vi "Find&Exchange_dots_ID-6.vi"(4 "Track ID Arr IN":u16[](array[numeric]), 5 "Dot matrix (stat)":i16[][](array[numeric]), 6 "track ID IN":u16, 7 "(X,Y...) Tracks":dbl[][](array[numeric]), 8 "error IN":errorcluster, 9 "frame (col)":i32, 10 "index of \ndot in frame":i32, 11 "ID-dot matrix":u16[][](array[numeric])) -> (0 "error OUT":errorcluster, 1 "track ID OUT":u16, 2 "Track ID Arr OUT":u16[](array[numeric]), 3 "ID-dot matrix OUT":u16[][](array[numeric]))   [LabVIEW 2013]
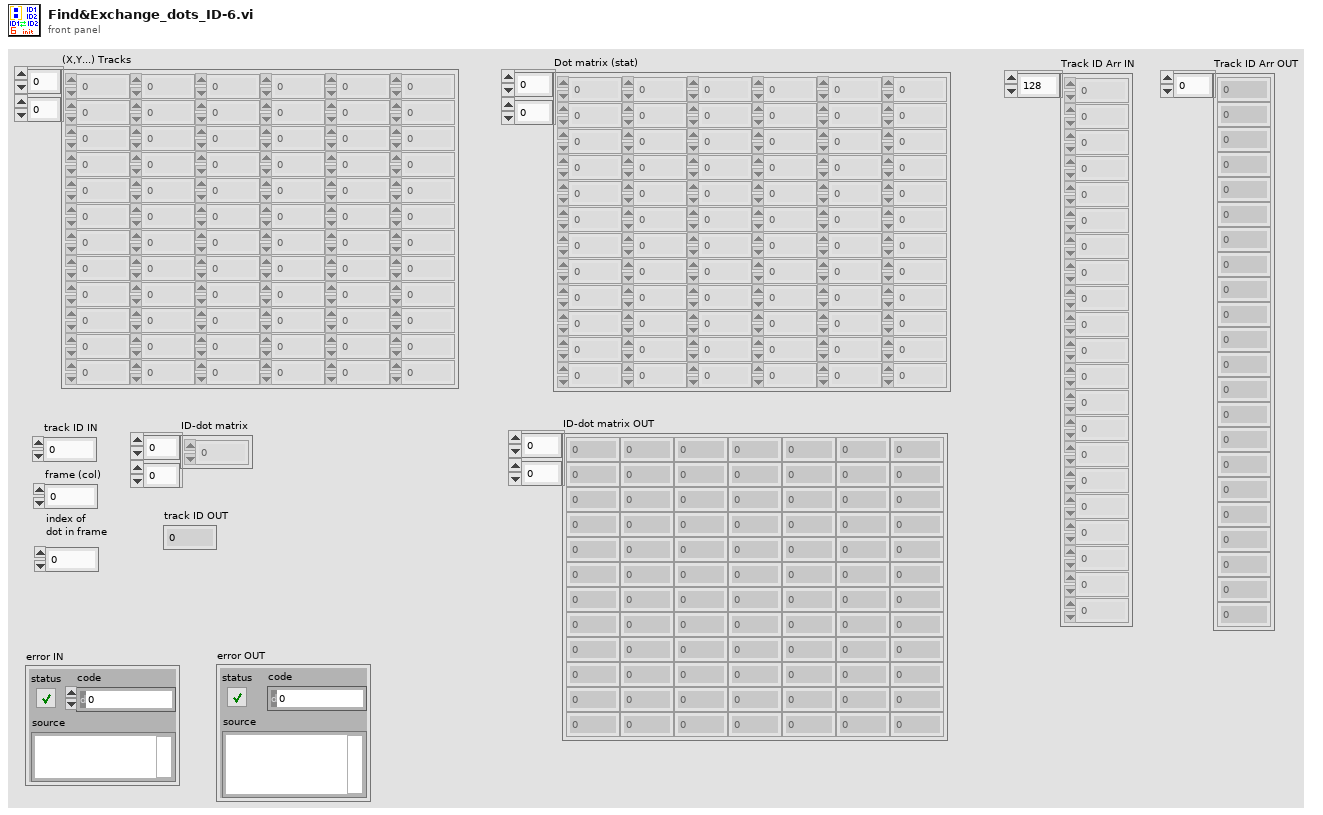
[diagram p1: front panel]
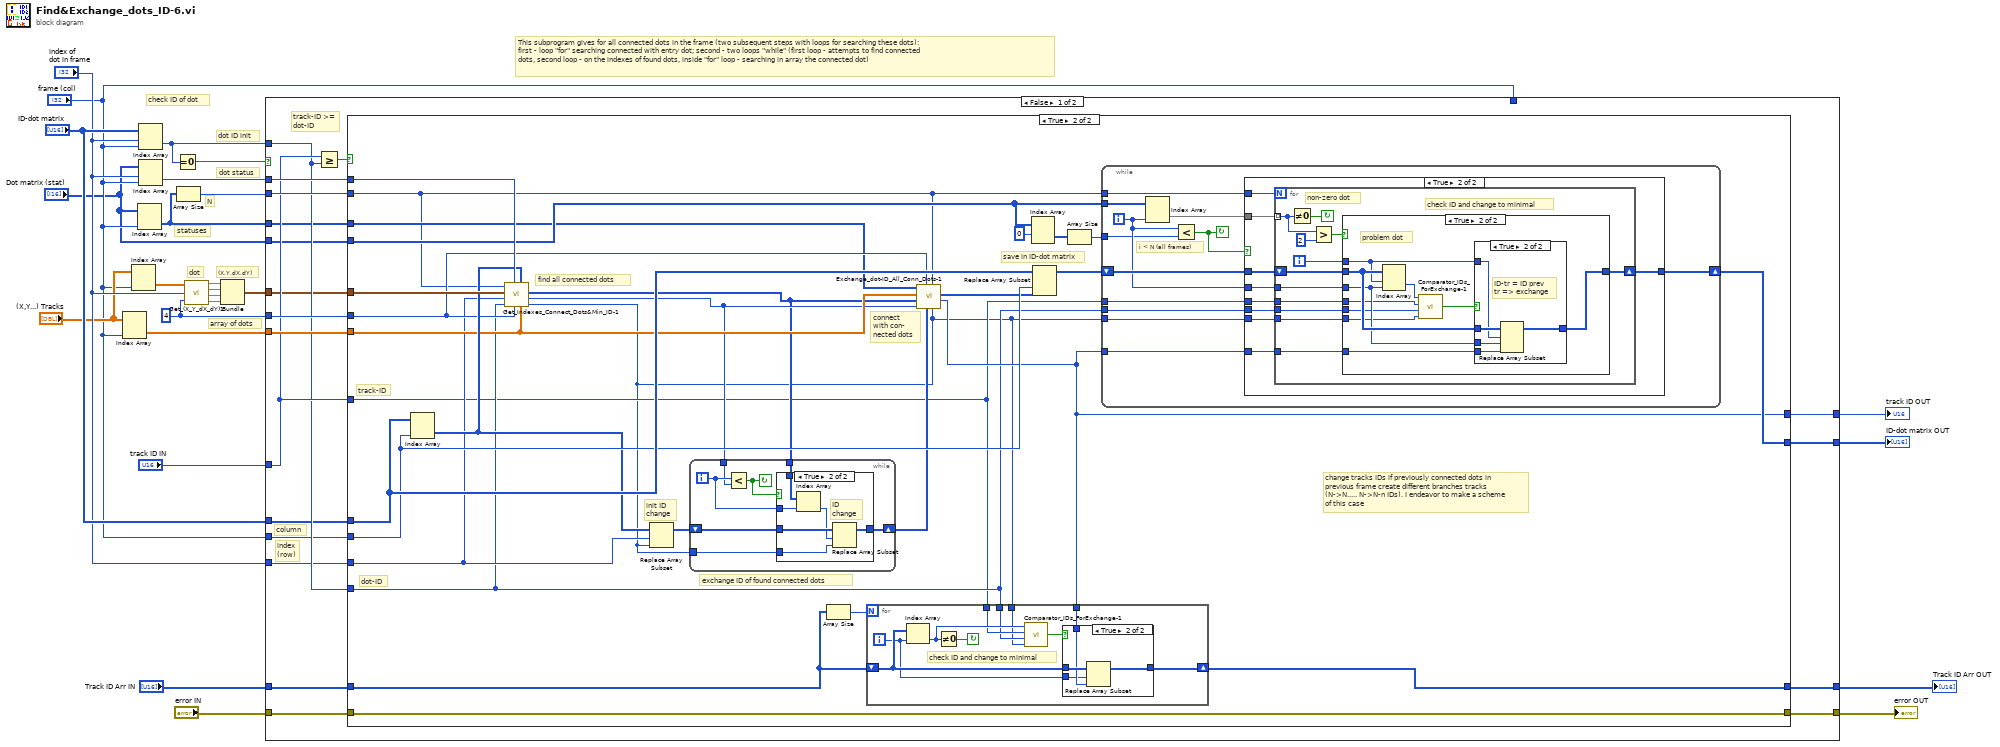
[diagram p0: block diagram]
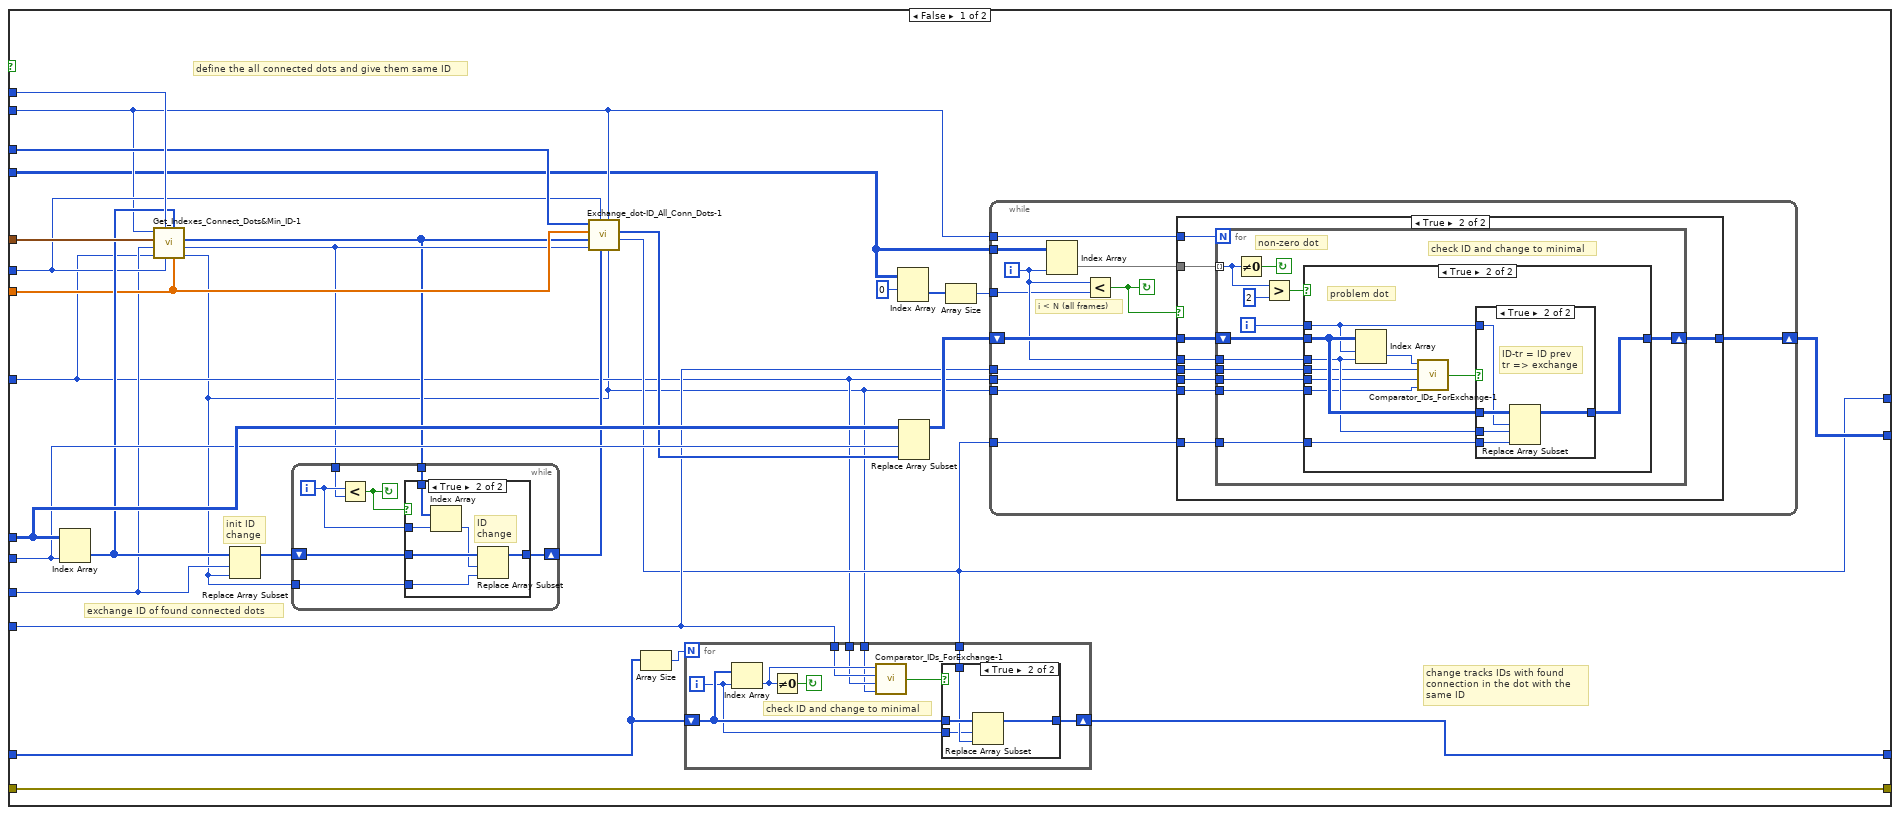
[diagram p2: hidden frame]
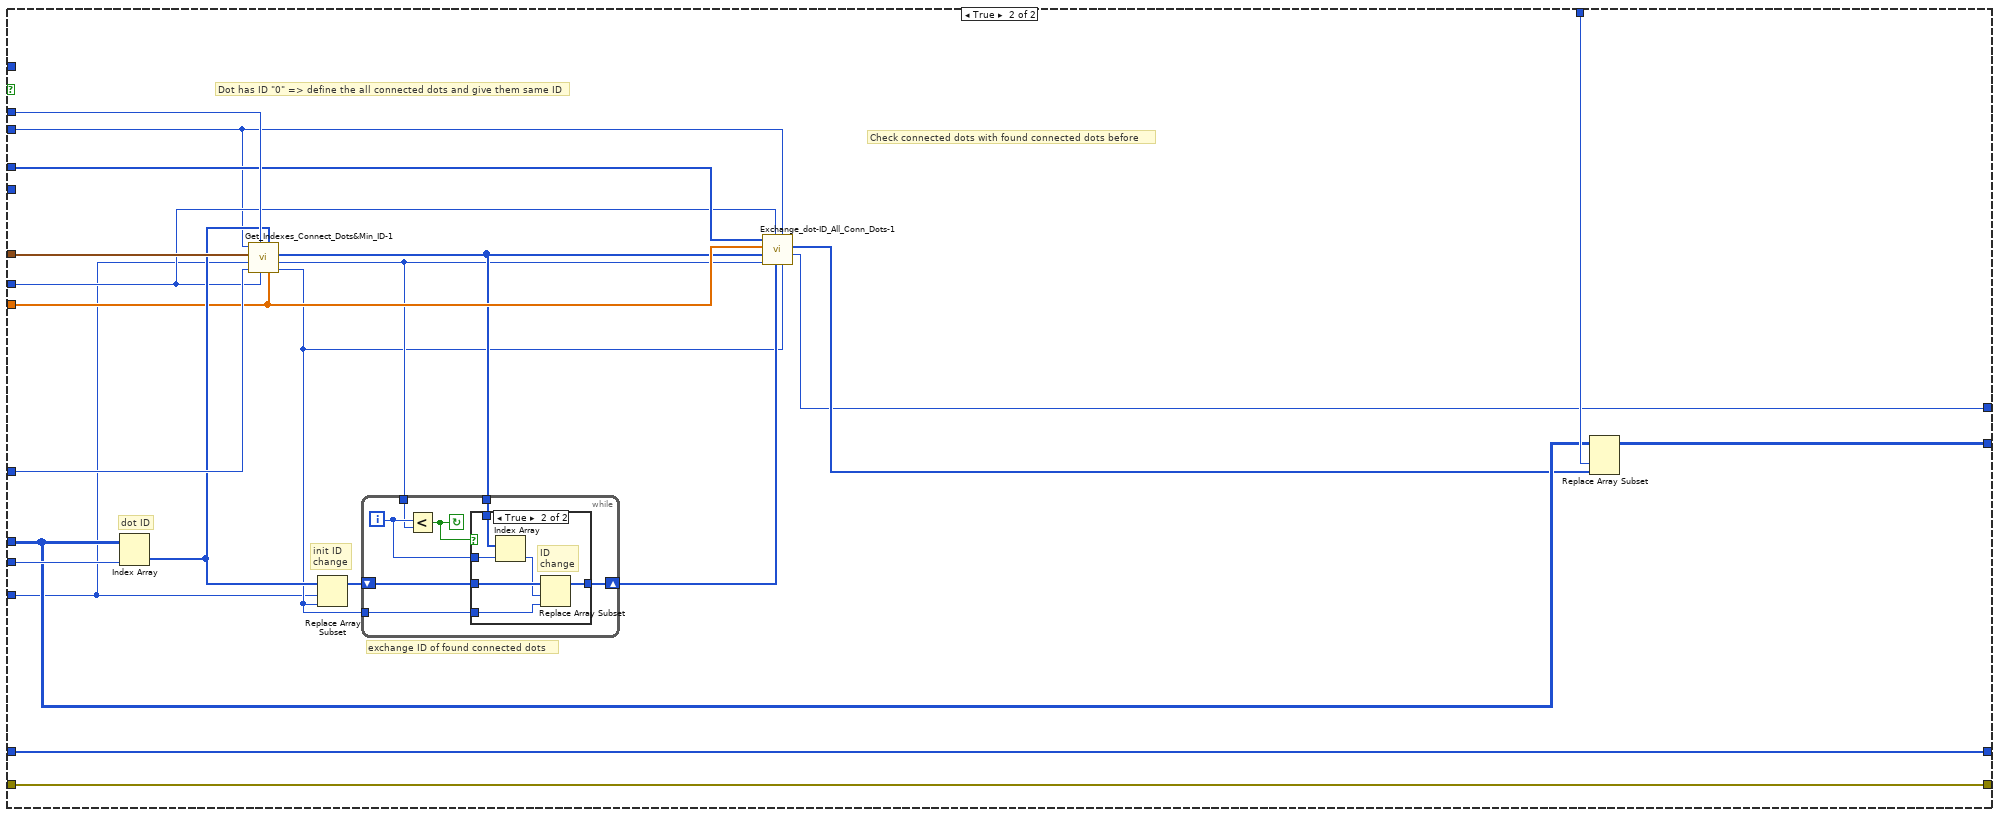
[diagram p13: hidden frame]
diagram:
  w19 = 4 ("multiplier")
  # "array of dots"
  # "dot ID init"
  # "dot status"
  # "(X,Y,dX,dY)"
  # "N"
  # "statuses"
  # "This subprogram gives for all connected dots in the frame (two subsequent steps with loops for searching these dots): \nfirst - loop \"for\" searching connected with entry dot; second - two loops \"while\" (first loop - attempts to find connected \ndots, second loop - on the indexes of found dots, inside \"for\" loop - searching in array the connected dot)"
  # "dot"
  # "check ID of dot"
  n1 = Index Array(array="(X,Y...) Tracks", index (col)="frame (col)") -> (element=w23:dbl[])  [unwired: 1 in]
  n2 = Index Array(array="(X,Y...) Tracks", index (col)="frame (col)") -> (element=w20:dbl[])  [unwired: 1 in]
  n3 = Index Array(array="Dot matrix (stat)", index (col)="frame (col)") -> (element=w24:i16[])  [unwired: 1 in]
  n4 = Index Array(array="ID-dot matrix", index (row)="index of \ndot in frame", index (col)="frame (col)") -> (element=w16:u16)
  n5 = Index Array(array="Dot matrix (stat)", index (row)="index of \ndot in frame", index (col)="frame (col)") -> (element=w22:i16)
  n6 = Equal To 0?(x=w16) -> (x = 0?=w21:bool)
  n7 = Array Size(array=w24) -> (size(s)=w25:i32)
  n8 = call "Get_(X_Y_dX_dY)1.vi"("(X,Y,dX,dY)"=w20, "index"="index of \ndot in frame", "multiplier"=w19) -> ("X"=w6:dbl, "Y"=w5:dbl, "dX"=w4:dbl, "dY"=w3:dbl)
  n9 = Bundle("X"=w6, "Y"=w5, "dX"=w4, "dY"=w3) -> (w2:cluster{"X":dbl, "Y":dbl, "dX":dbl, "dY":dbl})  [unwired: 1 in]
  n10 = case shown="False" w21 {
    tunnel: w25 -> [w39 w271]
    tunnel: w24 -> [w26 w273]
    tunnel: w23 -> [w38 w270]
    tunnel: w22 -> [w36 w276]
    tunnel: w19 -> [w37 w272]
    tunnel: "ID-dot matrix" -> [w32 w279]
    tunnel: "frame (col)" -> [w30 w280]
    tunnel: "index of \ndot in frame" -> [w28 w263]
    tunnel: "track ID IN" -> [w35 w275]
    tunnel: w16 -> [w34 _]
    tunnel: "error IN" -> [w43 w284]
    tunnel: [w42 w284] -> w13
    tunnel: [w41 w264] -> w12
    tunnel: [w31 w282] -> w11
    tunnel: "Track ID Arr IN" -> [w29 w281]
    tunnel: [w40 w281] -> w9
    tunnel: "frame (col)" -> [_ w283]
    tunnel: "Dot matrix (stat)" -> [w33 _]
    tunnel: w2 -> [w27 w277]
    frame False {
      # "column"
      # "index\n(row)"
      # "track-ID >=\ndot-ID"
      n11 = Greater Or Equal?(x=w35, y=w34) -> (x >= y?=w44:bool)
      n12 = case shown="True" w44 {
        tunnel: [w48 w166] -> w41
        tunnel: w34 -> [w50 w156]
        tunnel: w35 -> [w46 w155]
        tunnel: w43 -> [w71 w182]
        tunnel: [w71 w182] -> w42
        tunnel: w29 -> [w72 w180]
        tunnel: [w47 w179] -> w40
        tunnel: w39 -> [w52 w162]
        tunnel: w38 -> [w64 w164]
        tunnel: w37 -> [w63 w165]
        tunnel: w36 -> [w67 w173]
        tunnel: w33 -> [w51 w171]
        tunnel: w32 -> [w70 w178]
        tunnel: w30 -> [w69 w176]
        tunnel: [w49 w175] -> w31
        tunnel: w28 -> [w61 w161]
        tunnel: w27 -> [w68 w174]
        tunnel: w26 -> [w65 w163]
        frame False {
          # "define the all connected dots and give them same ID"
          # "init ID\nchange"
          # "exchange ID of found connected dots"
          # "change tracks IDs with found \nconnection in the dot with the \nsame ID"
          n13 = Index Array(array=w70, index (col)=w69) -> (element=w66:u16[])  [unwired: 1 in]
          n14 = call "Get_Indexes_Connect_Dots&Min_ID-1.vi"("(X,Y...) Tracks col"=w64, "ID-dot col"=w66, "multiplier (x4)"=w63, "dot status"=w67, "initial ID"=w46, "Current Dot \nindex"=w61, "Dot coord"=w68, "N elem. in col"=w52) -> ("minimal ID \nbetween them"=w45:u16, "amount"=w59:i32, "Indexex Connec\ndots"=w58:i32[])  [unwired: 1 in]
          n15 = Replace Array Subset(array=w66, new element=w45, index=w61) -> (w60:u16[])
          n16 = while {
            shift-right: [w129] -> w57
            shift-left: w60 -> [w128]
            tunnel: w45 -> [w127]
            tunnel: w59 -> [w125]
            tunnel: w58 -> [w130]
            i -> [w126]
            stop <- w131 continue-if-true
            n17 = Less?(x=w126, y=w125) -> (x < y?=w131:bool)
            n18 = case shown="True" w131 {
              tunnel: w130 -> [_ w138]
              tunnel: w126 -> [_ w137]
              tunnel: w128 -> [w132 w136]
              tunnel: w127 -> [_ w134]
              tunnel: [w132 w133] -> w129
              frame False {
              }
              frame True {
                # "ID\nchange"
                n19 = Index Array(array=w138, index=w137) -> (element=w135:i32)
                n20 = Replace Array Subset(array=w136, new element=w134, index=w135) -> (w133:u16[])
              }
            }
          }
          n21 = call "Exchange_dot-ID_All_Conn_Dots-1.vi"("Minimal ID"=w45, "N (all dots in frame)"=w52, "ID-dot col IN"=w57, "multiplier(x4)"=w63, "Amount"=w59, "Indexes Conn Dot"=w58, "(X,Y...)-col"=w64, "Statuses (col)"=w65) -> ("Minimal ID OUT"=w48:u16, "ID-dot col OUT"=w62:u16[])  [unwired: 2 in]
          n22 = Array Size(array=w72) -> (size(s)=w73:i32)
          n23 = for {
            N: w73 -> [_]
            shift-right: [w144] -> w47
            shift-left: w72 -> [w146]
            tunnel: w50 -> [w142]
            tunnel: w48 -> [w147]
            tunnel: w46 -> [w140]
            tunnel: w45 -> [w139]
            i -> [w145]
            stop <- w148 continue-if-true
            # "check ID and change to minimal"
            n24 = Index Array(array=w146, index=w145) -> (element=w143:u16)
            n25 = Not Equal To 0?(x=w143) -> (x != 0?=w148:bool)
            n26 = call "Comparator_IDs_ForExchange-1.vi"("Min ID Iter#1"=w139, "Initial ID"=w140, "Biggest ID (init)"=w142, "Current ID"=w143) -> ("ID = old ID"=w141:bool)
            n27 = case shown="True" w141 {
              tunnel: w147 -> [_ w152]
              tunnel: w146 -> [w149 w153]
              tunnel: w145 -> [_ w151]
              tunnel: [w149 w150] -> w144
              frame False {
              }
              frame True {
                n28 = Replace Array Subset(array=w153, new element=w152, index=w151) -> (w150:u16[])
              }
            }
          }
          n29 = Index Array(array=w51, index (row)=0) -> (element=w55:i16[])  [unwired: 1 in]
          n30 = Replace Array Subset(array=w70, new element=w62, index (col)=w69) -> (w53:u16[][])  [unwired: 1 in]
          n31 = Array Size(array=w55) -> (size(s)=w54:i32)
          n32 = while {
            tunnel: w51 -> [w85]
            shift-right: [w79] -> w49
            shift-left: w53 -> [w83]
            tunnel: w46 -> [w81]
            tunnel: w48 -> [w80]
            tunnel: w52 -> [w78]
            tunnel: w54 -> [w77]
            tunnel: w50 -> [w75]
            tunnel: w45 -> [w74]
            i -> [w82]
            stop <- w76 continue-if-true
            # "i < N (all frames)"
            n33 = Index Array(array=w85, index (col)=w82) -> (element=w84:i16[])  [unwired: 1 in]
            n34 = Less?(x=w82, y=w77) -> (x < y?=w76:bool)
            n35 = case shown="True" w76 {
              tunnel: w84 -> [_ w95]
              tunnel: w83 -> [w86 w94]
              tunnel: w82 -> [_ w93]
              tunnel: w81 -> [_ w92]
              tunnel: w80 -> [_ w91]
              tunnel: [w86 w90] -> w79
              tunnel: w78 -> [_ w89]
              tunnel: w75 -> [_ w88]
              tunnel: w74 -> [_ w87]
              frame False {
              }
              frame True {
                n36 = for {
                  N: w89 -> [_]
                  tunnel: w95 -> [w106] mode=indexing
                  tunnel: w93 -> [w102]
                  tunnel: w92 -> [w100]
                  tunnel: w91 -> [w99]
                  shift-right: [w98] -> w90
                  shift-left: w94 -> [w103]
                  tunnel: w88 -> [w97]
                  tunnel: w87 -> [w96]
                  i -> [w101]
                  stop <- w107 continue-if-true
                  # "check ID and change to minimal"
                  # "non-zero dot"
                  n37 = Not Equal To 0?(x=w106) -> (x != 0?=w107:bool)
                  n38 = Greater?(x=w106, y=i16 2) -> (0:w104:bool)
                  n39 = case shown="True" w104 {
                    tunnel: w103 -> [w108 w118]
                    tunnel: w102 -> [_ w117]
                    tunnel: w101 -> [_ w116]
                    tunnel: w100 -> [_ w111]
                    tunnel: w99 -> [_ w115]
                    tunnel: [w108 w114] -> w98
                    tunnel: w97 -> [_ w110]
                    tunnel: w96 -> [_ w109]
                    frame False {
                    }
                    frame True {
                      # "problem dot"
                      n40 = Index Array(array=w118, index (row)=w116, index (col)=w117) -> (element=w113:u16)
                      n41 = call "Comparator_IDs_ForExchange-1.vi"("Min ID Iter#1"=w109, "Initial ID"=w111, "Biggest ID (init)"=w110, "Current ID"=w113) -> ("ID = old ID"=w112:bool)
                      n42 = case shown="True" w112 {
                        tunnel: w118 -> [w119 w124]
                        tunnel: w117 -> [_ w123]
                        tunnel: w116 -> [_ w122]
                        tunnel: w115 -> [_ w121]
                        tunnel: [w119 w120] -> w114
                        frame False {
                        }
                        frame True {
                          # "ID-tr = ID prev \ntr => exchange"
                          n43 = Replace Array Subset(array=w124, new element=w121, index (row)=w122, index (col)=w123) -> (w120:u16[][])
                        }
                      }
                    }
                  }
                }
              }
            }
          }
        }
        frame True {
          # "save in ID-dot matrix"
          # "connect\nwith con-\nnected dots"
          # "find all connected dots"
          # "dot-ID"
          # "track-ID"
          # "init ID\nchange"
          # "exchange ID of found connected dots"
          # "change tracks IDs if previously connected dots in \nprevious frame create different branches tracks\n(N->N..... N->N-n IDs). I endeavor to make a scheme\nof this case"
          n44 = Index Array(array=w178, index (col)=w176) -> (element=w172:u16[])  [unwired: 1 in]
          n45 = call "Get_Indexes_Connect_Dots&Min_ID-1.vi"("(X,Y...) Tracks col"=w164, "ID-dot col"=w172, "multiplier (x4)"=w165, "dot status"=w173, "initial ID"=w156, "Current Dot \nindex"=w161, "Dot coord"=w174, "N elem. in col"=w162) -> ("minimal ID \nbetween them"=w154:u16, "amount"=w160:i32, "Indexex Connec\ndots"=w159:i32[])  [unwired: 1 in]
          n46 = Replace Array Subset(array=w172, new element=w154, index=w161) -> (w157:u16[])
          n47 = while {
            shift-right: [w187] -> w158
            shift-left: w157 -> [w186]
            tunnel: w154 -> [w185]
            tunnel: w160 -> [w183]
            tunnel: w159 -> [w188]
            i -> [w184]
            stop <- w189 continue-if-true
            n48 = Less?(x=w184, y=w183) -> (x < y?=w189:bool)
            n49 = case shown="True" w189 {
              tunnel: w188 -> [_ w196]
              tunnel: w184 -> [_ w195]
              tunnel: w186 -> [w190 w194]
              tunnel: w185 -> [_ w192]
              tunnel: [w190 w191] -> w187
              frame False {
              }
              frame True {
                # "ID\nchange"
                n50 = Index Array(array=w196, index=w195) -> (element=w193:i32)
                n51 = Replace Array Subset(array=w194, new element=w192, index=w193) -> (w191:u16[])
              }
            }
          }
          n52 = Array Size(array=w180) -> (size(s)=w181:i32)
          n53 = call "Exchange_dot-ID_All_Conn_Dots-1.vi"("Minimal ID"=w154, "N (all dots in frame)"=w162, "ID-dot col IN"=w158, "multiplier(x4)"=w165, "Amount"=w160, "Indexes Conn Dot"=w159, "(X,Y...)-col"=w164, "Statuses (col)"=w163) -> ("Minimal ID OUT"=w166:u16, "ID-dot col OUT"=w167:u16[])  [unwired: 2 in]
          n54 = for {
            N: w181 -> [_]
            shift-right: [w253] -> w179
            shift-left: w180 -> [w255]
            tunnel: w155 -> [w251]
            tunnel: w166 -> [w256]
            tunnel: w156 -> [w250]
            tunnel: w154 -> [w249]
            i -> [w254]
            stop <- w257 continue-if-true
            # "check ID and change to minimal"
            n55 = Index Array(array=w255, index=w254) -> (element=w252:u16)
            n56 = Not Equal To 0?(x=w252) -> (x != 0?=w257:bool)
            n57 = call "Comparator_IDs_ForExchange-1.vi"("Min ID Iter#1"=w249, "Initial ID"=w250, "Biggest ID (init)"=w251, "Current ID"=w252) -> ("ID = old ID"=w248:bool)
            n58 = case shown="True" w248 {
              tunnel: w256 -> [_ w261]
              tunnel: w255 -> [w258 w262]
              tunnel: w254 -> [_ w260]
              tunnel: [w258 w259] -> w253
              frame False {
              }
              frame True {
                n59 = Replace Array Subset(array=w262, new element=w261, index=w260) -> (w259:u16[])
              }
            }
          }
          n60 = Index Array(array=w171, index (row)=0) -> (element=w169:i16[])  [unwired: 1 in]
          n61 = Replace Array Subset(array=w178, new element=w167, index (col)=w176) -> (w177:u16[][])  [unwired: 1 in]
          n62 = Array Size(array=w169) -> (size(s)=w168:i32)
          n63 = while {
            tunnel: w171 -> [w208]
            shift-right: [w203] -> w175
            shift-left: w177 -> [w206]
            tunnel: w166 -> [w204]
            tunnel: w162 -> [w202]
            tunnel: w168 -> [w201]
            tunnel: w156 -> [w199]
            tunnel: w155 -> [w198]
            tunnel: w154 -> [w197]
            i -> [w205]
            stop <- w200 continue-if-true
            # "i < N (all frames)"
            n64 = Index Array(array=w208, index (col)=w205) -> (element=w207:i16[])  [unwired: 1 in]
            n65 = Less?(x=w205, y=w201) -> (x < y?=w200:bool)
            n66 = case shown="True" w200 {
              tunnel: w207 -> [_ w218]
              tunnel: w206 -> [w209 w217]
              tunnel: w205 -> [_ w216]
              tunnel: w204 -> [_ w215]
              tunnel: [w209 w214] -> w203
              tunnel: w202 -> [_ w213]
              tunnel: w199 -> [_ w212]
              tunnel: w198 -> [_ w211]
              tunnel: w197 -> [_ w210]
              frame False {
              }
              frame True {
                n67 = for {
                  N: w213 -> [_]
                  tunnel: w218 -> [w229] mode=indexing
                  tunnel: w216 -> [w225]
                  tunnel: w215 -> [w223]
                  shift-right: [w222] -> w214
                  shift-left: w217 -> [w226]
                  tunnel: w212 -> [w221]
                  tunnel: w211 -> [w220]
                  tunnel: w210 -> [w219]
                  i -> [w224]
                  stop <- w230 continue-if-true
                  # "check ID and change to minimal"
                  # "non-zero dot"
                  n68 = Not Equal To 0?(x=w229) -> (x != 0?=w230:bool)
                  n69 = Greater?(x=w229, y=i16 2) -> (0:w227:bool)
                  n70 = case shown="True" w227 {
                    tunnel: w226 -> [w231 w241]
                    tunnel: w225 -> [_ w240]
                    tunnel: w224 -> [_ w239]
                    tunnel: w223 -> [_ w238]
                    tunnel: [w231 w237] -> w222
                    tunnel: w221 -> [_ w235]
                    tunnel: w220 -> [_ w232]
                    tunnel: w219 -> [_ w234]
                    frame False {
                    }
                    frame True {
                      # "problem dot"
                      n71 = Index Array(array=w241, index (row)=w239, index (col)=w240) -> (element=w236:u16)
                      n72 = call "Comparator_IDs_ForExchange-1.vi"("Min ID Iter#1"=w234, "Initial ID"=w235, "Biggest ID (init)"=w232, "Current ID"=w236) -> ("ID = old ID"=w233:bool)
                      n73 = case shown="True" w233 {
                        tunnel: w241 -> [w242 w247]
                        tunnel: w240 -> [_ w246]
                        tunnel: w239 -> [_ w245]
                        tunnel: w238 -> [_ w244]
                        tunnel: [w242 w243] -> w237
                        frame False {
                        }
                        frame True {
                          # "ID-tr = ID prev \ntr => exchange"
                          n74 = Replace Array Subset(array=w247, new element=w244, index (row)=w245, index (col)=w246) -> (w243:u16[][])
                        }
                      }
                    }
                  }
                }
              }
            }
          }
        }
      }
    }
    frame True {
      # "Check connected dots with found connected dots before"
      # "Dot has ID \"0\" => define the all connected dots and give them same ID"
      # "init ID\nchange"
      # "exchange ID of found connected dots"
      # "dot ID"
      n75 = Index Array(array=w279, index (col)=w280) -> (element=w274:u16[])  [unwired: 1 in]
      n76 = call "Get_Indexes_Connect_Dots&Min_ID-1.vi"("(X,Y...) Tracks col"=w270, "ID-dot col"=w274, "multiplier (x4)"=w272, "dot status"=w276, "initial ID"=w275, "Current Dot \nindex"=w263, "Dot coord"=w277, "N elem. in col"=w271) -> ("minimal ID \nbetween them"=w266:u16, "amount"=w268:i32, "Indexex Connec\ndots"=w269:i32[])  [unwired: 1 in]
      n77 = Replace Array Subset(array=w274, new element=w266, index=w263) -> (w278:u16[])
      n78 = while {
        shift-right: [w289] -> w267
        shift-left: w278 -> [w288]
        tunnel: w266 -> [w287]
        tunnel: w268 -> [w285]
        tunnel: w269 -> [w290]
        i -> [w286]
        stop <- w291 continue-if-true
        n79 = Less?(x=w286, y=w285) -> (x < y?=w291:bool)
        n80 = case shown="True" w291 {
          tunnel: w290 -> [_ w298]
          tunnel: w286 -> [_ w297]
          tunnel: w288 -> [w292 w296]
          tunnel: w287 -> [_ w294]
          tunnel: [w292 w293] -> w289
          frame False {
          }
          frame True {
            # "ID\nchange"
            n81 = Index Array(array=w298, index=w297) -> (element=w295:i32)
            n82 = Replace Array Subset(array=w296, new element=w294, index=w295) -> (w293:u16[])
          }
        }
      }
      n83 = call "Exchange_dot-ID_All_Conn_Dots-1.vi"("Minimal ID"=w266, "N (all dots in frame)"=w271, "ID-dot col IN"=w267, "multiplier(x4)"=w272, "Amount"=w268, "Indexes Conn Dot"=w269, "(X,Y...)-col"=w270, "Statuses (col)"=w273) -> ("Minimal ID OUT"=w264:u16, "ID-dot col OUT"=w265:u16[])  [unwired: 2 in]
      n84 = Replace Array Subset(array=w279, new element=w265, index (col)=w283) -> (w282:u16[][])  [unwired: 1 in]
    }
  }
  "error OUT" <- w13
  "ID-dot matrix OUT" <- w11
  "track ID OUT" <- w12
  "Track ID Arr OUT" <- w9
